vi "SetSBEventDataHelper.vi"(10 "SearchBrowser":T1) -> (2 "SearchBrowser":T1)   [LabVIEW 2014, in "FRCts20_EspEngine.lvlib"]
uses:
  FRCts20_EspEngine.lvlib
  TypeDefs/FRCts20_EspEngine_SearchBrowser.ctl
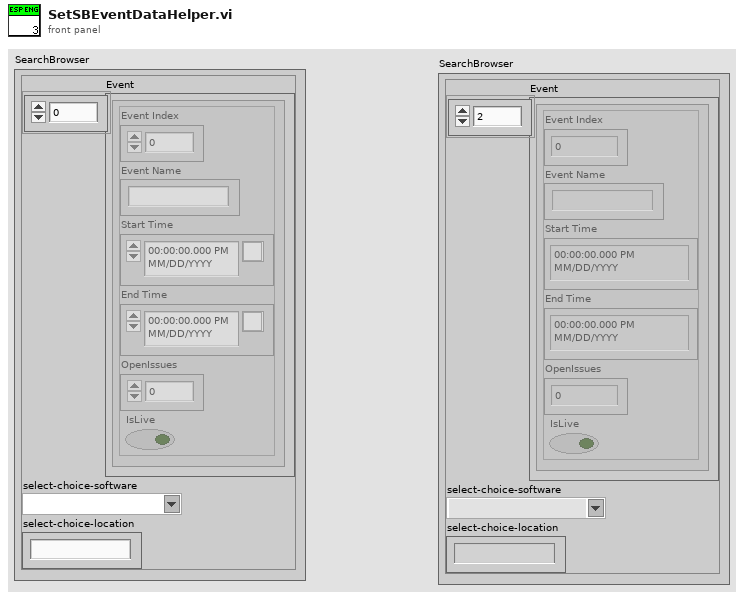
[diagram p1: front panel]
types:
  T1 = typedef "FRCts20_EspEngine.lvlib/FRCts20_EspEngine_SearchBrowser.ctl" = cluster{"Event":cluster{"Event Index":u32, "Event Name":string, "Start Time":timestamp, "End Time":timestamp, "OpenIssues":u8, "IsLive":bool}[], "select-choice-software":string, "select-choice-location":string}
  T2 = cluster{"Event Index":u32, "Event Name":string, "Start Time":timestamp, "End Time":timestamp, "OpenIssues":u8, "IsLive":bool}[]
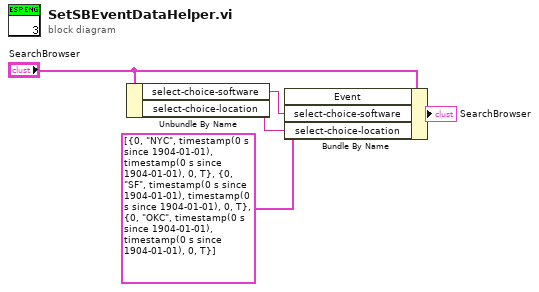
[diagram p0: block diagram]
diagram:
  n1 = Unbundle By Name("SearchBrowser") -> ("select-choice-software"=w4:string, "select-choice-location"=w3:string)
  n2 = Bundle By Name(cluster="SearchBrowser", "Event"=T2 [{"Event Index"=0, "Event Name"="NYC", "Start Time"=timestamp(0 s since 1904-01-01), "End Time"=timestamp(0 s since 1904-01-01), "OpenIssues"=0, "IsLive"=TRUE}, {"Event Index"=0, "Event Name"="SF", "Start Time"=timestamp(0 s since 1904-01-01), "End Time"=timestamp(0 s since 1904-01-01), "OpenIssues"=0, "IsLive"=TRUE}, {"Event Index"=0, "Event Name"="OKC", "Start Time"=timestamp(0 s since 1904-01-01), "End Time"=timestamp(0 s since 1904-01-01), "OpenIssues"=0, "IsLive"=TRUE}], "select-choice-software"=w4, "select-choice-location"=w3) -> (→"SearchBrowser":T1)
